vi "PLC_to_Auto.vi"() -> ()   [LabVIEW 2017]
panel:
  out "MOTOR PARAMETER":bool
  in  "scanner data":string
  out "AUTO SCREEN ON":bool
  out "I/O MANUAL ON":bool
  out "I/O SCREEN ON":bool
  out "PLC Communication STATION 1":bool
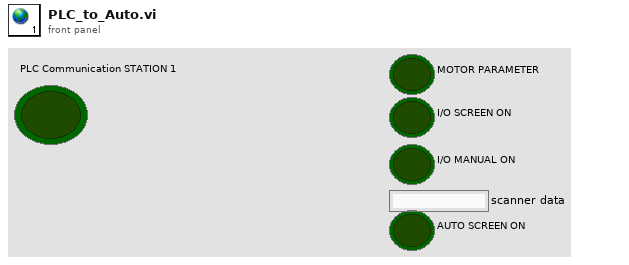
[diagram p1: front panel]
diagram:
